vi "Enqueue Element.vi"(8 "error in":errorcluster, 11 "Message":T1) -> (0 "error out":errorcluster)   [LabVIEW 2018, in "Template Module.lvlib"]
doc: "Enqueues element"
uses:
  Template Module.lvlib
  ctl/Message--enum.ctl
  ctl/State--enum.ctl
  ctl/Queue action--enum.ctl
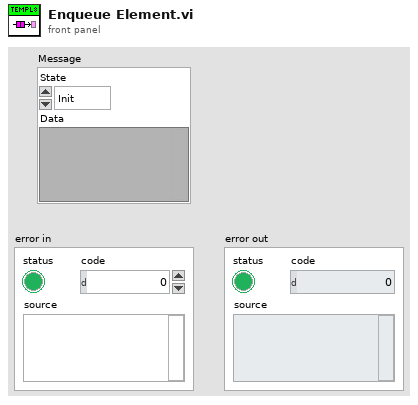
[diagram p1: front panel]
types:
  T1 = typedef "Template Module.lvlib/Message--enum.ctl" = cluster{"State":T2, "Data":variant}
  T2 = typedef "Template Module.lvlib/State--enum.ctl" = enum16{"Init", "Error", "Close"}
  T3 = typedef "Template Module.lvlib/Queue action--enum.ctl" = enum16{"Create", "Get", "Destroy"}
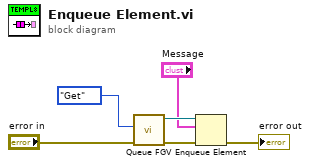
[diagram p0: block diagram]
diagram:
  n1 = call "Queue FGV.vi"("error in"="error in", "Queue Action"=Queue_action--enum."Get") -> ("error out"=w2:errorcluster, "Queue reference"=w3:refnum<queue>)  [unwired: 8 in]
  n2 = Enqueue Element(queue=w3, element="Message", error in (no error)=w2) -> (error out=→"error out":errorcluster)  [unwired: 1 in, 2 out]
